vi "获取运行状态.vi"(8 "error in (no error)":errorcluster) -> (0 "error out":errorcluster, 1 "堵转偏差值":u16, 2 "字状态":T1, 3 "位状态":T2)   [LabVIEW 2016, in "PLC.lvlib"]
uses:
  PLC.lvlib
  <vilib>/Plasmionique/MB Master/MB_Master_Serial/MB_Master_Serial.lvclass
  C:/Program Files (x86)/National Instruments/LabVIEW 2016/vi.lib/Plasmionique/MB Master/MB_Master/MB_Master.lvclass
  <vilib>/Plasmionique/MB Master/MB Master.lvlib
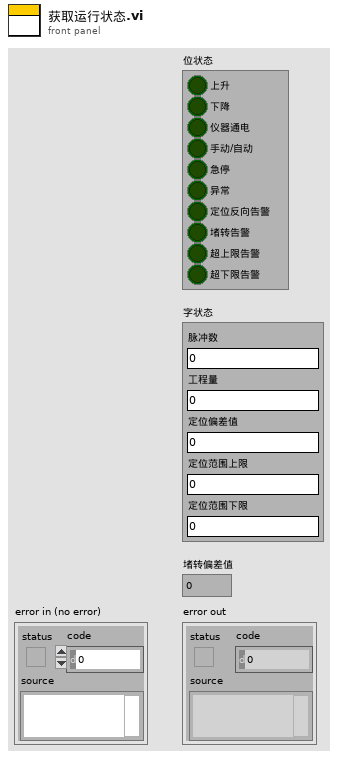
[diagram p1: front panel]
types:
  T1 = cluster{"脉冲数":sgl, "工程量":sgl, "定位偏差值":sgl, "定位范围上限":sgl, "定位范围下限":sgl}
  T2 = cluster{"上升":bool, "下降":bool, "仪器通电":bool, "手动/自动":bool, "急停":bool, "异常":bool, "定位反向告警":bool, "堵转告警":bool, "超上限告警":bool, "超下限告警":bool}
  T3 = cluster{"Coils[0]":bool, "Coils[1]":bool, "Coils[2]":bool, "Coils[3]":bool, "Coils[4]":bool, "Coils[5]":bool, "Coils[6]":bool, "Coils[7]":bool, "Coils[8]":bool, "Coils[9]":bool}
  T4 = cluster{"[0]":sgl, "[1]":sgl, "[2]":sgl, "[3]":sgl, "[4]":sgl}
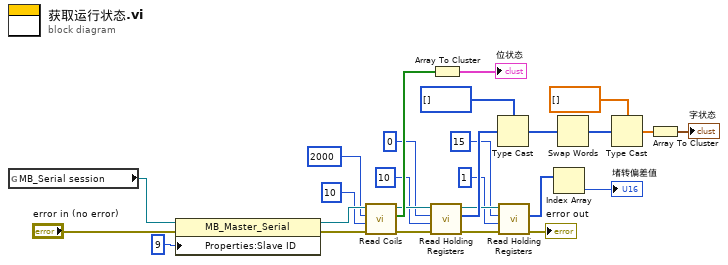
[diagram p0: block diagram]
diagram:
  n1 = global read "中间变量.vi" "MB_Serial session"() -> (w27:refnum<class "MB_Master_Serial.lvclass">)
  n2 = property class="MB_Master_Serial"(reference=w27, error in="error in (no error)", "Properties:Slave ID"=u8 9 ("Slave ID")) -> (reference out=w26:refnum<class "MB_Master_Serial.lvclass">, error out=w23:errorcluster)
  n3 = call <vilib>:"Read Coils.vi"("error in (no error)"=w23, "quantity"=u16 10, "starting address"=u16 2000, "MB session in"=w26) -> ("error out"=w17:errorcluster, "Coils"=w20:bool[], "MB session out"=w18:refnum<class "MB_Master_Serial.lvclass">)  [unwired: 5 in]
  n4 = call <vilib>:"Read Holding Registers.vi"("error in (no error)"=w17, "quantity"=u16 10, "starting address"=u16 0, "MB session in"=w18) -> ("error out"=w6:errorcluster, "Registers"=w14:u16[], "MB session out"=w7:refnum<class "MB_Master_Serial.lvclass">)  [unwired: 5 in]
  n5 = Array To Cluster(array=w20) -> (cluster=→"位状态":T3)
  n6 = Type Cast(type=i32[] [], x=w14) -> (*(type *) &x=w12:i32[])
  n7 = call <vilib>:"Read Holding Registers.vi"("error in (no error)"=w6, "quantity"=u16 1, "starting address"=u16 15, "MB session in"=w7) -> ("error out"=→"error out":errorcluster, "Registers"=w3:u16[])  [unwired: 5 in, 1 out]
  n8 = Index Array(array=w3) -> (element=→"堵转偏差值":u16)  [unwired: 1 in]
  n9 = Swap Words(1:w12) -> (0:w11:i32[])
  n10 = Type Cast(type=sgl[] [], x=w11) -> (*(type *) &x=w9:sgl[])
  n11 = Array To Cluster(array=w9) -> (cluster=→"字状态":T4)
